vi "compatReadText.vi"(5 "convert eol (F)":bool, 6 "count":i32, 7 "line mode (F)":bool, 8 "error in":errorcluster, 11 "refnum":refnum<file>) -> (0 "error out":errorcluster, 2 "data":string, 3 "dup refnum":refnum<file>)   [LabVIEW 2015]
doc: "Compatibility VI to preserve functionality of the LabVIEW 7.1 Read File primitive."
panel:
  # "This VI should only be used when nothing was connected to byte stream type,\nand at least one of line mode or convert eol was wired."
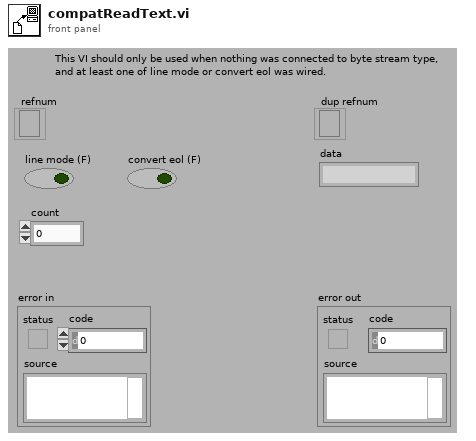
[diagram p1: front panel]
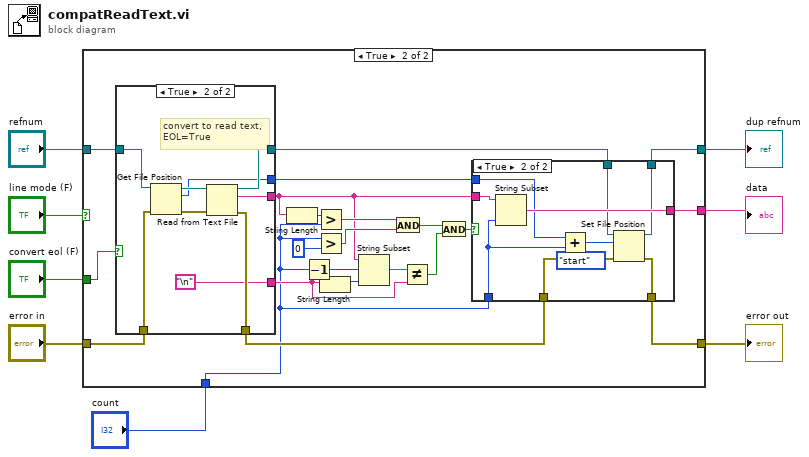
[diagram p0: block diagram]
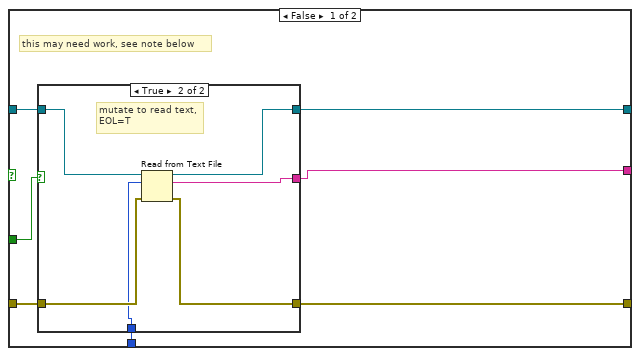
[diagram p2: hidden frame]
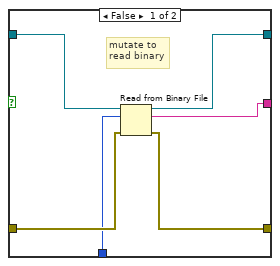
[diagram p3: hidden frame]
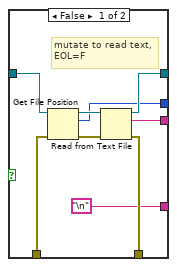
[diagram p5: hidden frame]
diagram:
  n1 = case shown="True" "line mode (F)" {
    tunnel: [w12 w41] -> w7
    tunnel: "refnum" -> [w13 w49]
    tunnel: "error in" -> [w15 w48]
    tunnel: [w14 w39] -> w5
    tunnel: "count" -> [w11 w29]
    tunnel: [w10 w43] -> w3
    tunnel: "convert eol (F)" -> [w9 w47]
    frame False {
      # "this may need work, see note below"
      n2 = case shown="True" w9 {
        tunnel: w15 -> [w17 w24]
        tunnel: [w18 w25] -> w14
        tunnel: [w21 w27] -> w12
        tunnel: w13 -> [w20 w22]
        tunnel: w11 -> [w16 w23]
        tunnel: [w19 w26] -> w10
        frame False {
          # "mutate to\nread binary"
          n3 = Read from Binary File(8:w17, 10:w16, 11:w20) -> (0:w18:errorcluster, 2:w19:string, 3:w21:refnum<file>)  [unwired: 3 in, 1 out]
        }
        frame True {
          # "mutate to read text,\nEOL=T"
          n4 = Read from Text File(file (use dialog)=w22, count=w23, error in=w24) -> (refnum out=w27:refnum<file>, text=w26:string, error out=w25:errorcluster)  [unwired: 1 in, 1 out]
        }
      }
    }
    frame True {
      n5 = case shown="True" w47 {
        tunnel: w49 -> [w66 w74]
        tunnel: w48 -> [w65 w75]
        tunnel: [w71 w80] -> w40
        tunnel: [w70 w79] -> w42
        tunnel: [w69 w78] -> w34
        tunnel: [w64 w73] -> w38
        tunnel: ["\n" "\n"] -> w33
        frame False {
          # "mutate to read text,\nEOL=F"
          n6 = Get File Position(4:w65, 7:w66) -> (0:w68:errorcluster, 2:w64:i64, 3:w67:refnum<file>)
          n7 = Read from Text File(file (use dialog)=w67, error in=w68) -> (refnum out=w70:refnum<file>, text=w69:string, error out=w71:errorcluster)  [unwired: 2 in, 1 out]
        }
        frame True {
          # "convert to read text,\nEOL=True"
          n8 = Get File Position(4:w75, 7:w74) -> (0:w77:errorcluster, 2:w73:i64, 3:w76:refnum<file>)
          n9 = Read from Text File(file (use dialog)=w76, error in=w77) -> (refnum out=w79:refnum<file>, text=w78:string, error out=w80:errorcluster)  [unwired: 2 in, 1 out]
        }
      }
      n10 = String Length(string=w34) -> (length=w44:i32)
      n11 = Decrement(x=w29) -> (x-1=w28:i32)
      n12 = Greater?(x=w44, y=w29) -> (0:w45:bool)
      n13 = Greater?(x=w29, y=0) -> (0:w46:bool)
      n14 = String Length(string=w33) -> (length=w35:i32)
      n15 = String Subset(string=w34, offset (0)=w28, length (rest)=w35) -> (substring=w32:string)
      n16 = And(x=w45, y=w46) -> (x .and. y?=w37:bool)
      n17 = Not Equal?(x=w32, y=w33) -> (x != y?=w31:bool)
      n18 = And(x=w37, y=w31) -> (x .and. y?=w36:bool)
      n19 = case shown="True" w36 {
        tunnel: [w52 w62] -> w43
        tunnel: w34 -> [w52 w61]
        tunnel: w29 -> [_ w58]
        tunnel: w42 -> [w51 w54]
        tunnel: [w51 w60] -> w41
        tunnel: w40 -> [w50 w55]
        tunnel: [w50 w59] -> w39
        tunnel: w38 -> [_ w56]
        frame False {
        }
        frame True {
          n20 = String Subset(string=w61, length (rest)=w58) -> (substring=w62:string)  [unwired: 1 in]
          n21 = Add(x=w56, y=w58) -> (x+y=w57:i64)
          n22 = Set File Position(offset (in bytes) (0)=w57, refnum=w54, from (0:start)=enum16{"start", "end", "current"}."start", error in=w55) -> (refnum out=w60:refnum<file>, error out=w59:errorcluster)
        }
      }
    }
  }
  "error out" <- w5
  "data" <- w3
  "dup refnum" <- w7
